vi "UART Read.vi"() -> ()   [LabVIEW 2020, in "CTI-Visa-Scratchpad.lvlib"]
uses:
  CTI-Visa-Scratchpad.lvlib
  CTI-Visa/CTI-Visa.lvlib
panel:
  out "String":string
  in  "stop":bool
  in  "RX GPIO":u8=9
  in  "TX GPIO":u8=8
  in  "Baud":u32=9600
  in  "UART":u8=1
  in  "Port":refnum<visa-resource-name>="COM3"
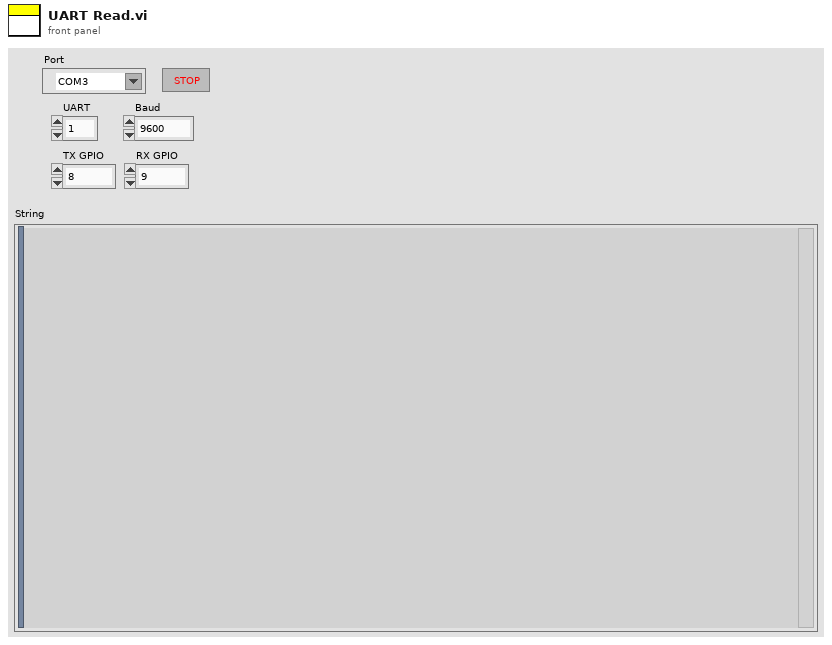
[diagram p1: front panel]
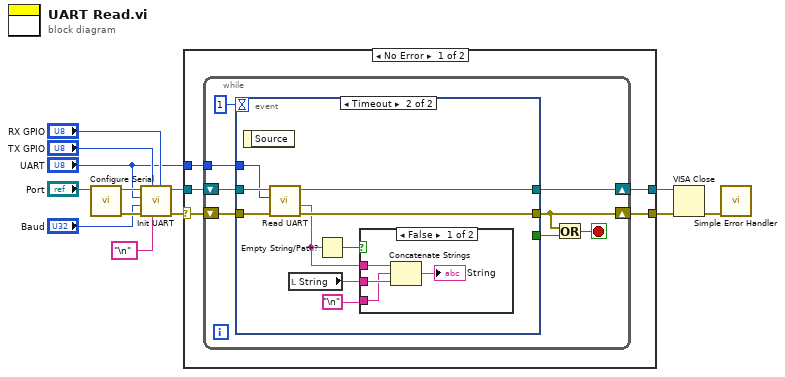
[diagram p0: block diagram]
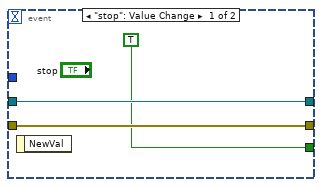
[diagram p2: hidden frame]
diagram:
  n1 = call "Configure Serial.vi"("VISA resource name in"="Port") -> ("error out"=w9:errorcluster, "VISA resource name"=w12:refnum<visa-resource-name>)  [unwired: 9 in]
  n2 = call "Init UART.vi"("RX GPIO"="RX GPIO", "Term Char (None)"="\n", "TX GPIO"="TX GPIO", "error in (no error)"=w9, "Baud"="Baud", "UART"="UART", "VISA resource name in"=w12) -> ("error out"=w7:errorcluster, "VISA resource name"=w6:refnum<visa-resource-name>)  [unwired: 3 in]
  n3 = case shown="No Error" w7 {
    selector: w7 -> [w16 w44]
    tunnel: w6 -> [w17 w43]
    tunnel: "UART" -> [w18 _]
    tunnel: [w15 w44] -> w4
    tunnel: [w14 w43] -> w3
    frame No Error {
      n4 = while {
        tunnel: w18 -> [w25]
        shift-right: [w24] -> w14
        shift-left: w17 -> [w26]
        shift-right: [w22] -> w15
        shift-left: w16 -> [w23]
        stop <- w20 stop-if-true
        n5 = event shown="[1] Timeout" {
          selector: _ -> [_ _]
          dyn-events: _ -> [_ _]
          timeout: 1 -> [_ _]
          tunnel: w26 -> [w29 w38]
          tunnel: w25 -> [_ w36]
          tunnel: [w29 w34] -> w24
          tunnel: w23 -> [w28 w37]
          tunnel: [w28 w35] -> w22
          tunnel: [TRUE _] -> w21
          event "stop": Value Change {
            n6 = event-data() -> ()  [unwired: 1 in, 1 out]
          }
          event Timeout {
            n7 = event-data() -> ()  [unwired: 1 in, 1 out]
            n8 = call "Read UART.vi"("error in (no error)"=w37, "UART"=w36, "VISA resource name in"=w38) -> ("error out"=w35:errorcluster, "Data"=w30:string, "VISA resource name"=w34:refnum<visa-resource-name>)  [unwired: 6 in]
            n9 = local read "String"() -> (w33:string)
            n10 = Empty String/Path?(string/path=w30) -> (empty?=w32:bool)
            n11 = case shown="False" w32 {
              tunnel: w33 -> [w42 _]
              tunnel: w30 -> [w41 _]
              tunnel: "\n" -> [w39 _]
              frame False {
                n12 = Concatenate Strings(w41, w39, w42) -> (→"String":string)
              }
              frame True {
              }
            }
          }
        }
        n13 = Or(x=w22, y=w21) -> (x .or. y?=w20:bool)
      }
    }
    frame Error {
    }
  }
  n14 = VISA Close(VISA resource name=w3, error in (no error)=w4) -> (error out=w2:errorcluster)
  n15 = call <vilib>:"Simple Error Handler.vi"("error in (no error)"=w2) -> ()  [unwired: 4 in, 5 out]
